vi "terminate.vi"(8 "error in (no error)":errorcluster, 11 "GenericImageProcessor in":refnum<class "GenericImageProcessor.lvclass">) -> (0 "error out":errorcluster, 3 "GenericImageProcessor out":refnum<class "GenericImageProcessor.lvclass">)   [LabVIEW 2010, in "GenericImageProcessor.lvclass"]
uses:
  GenericImageProcessor.lvclass
  GenericImageProcessor.lvclass/GenericImageProcessor.ctl
  common/classes/Image/Image/Image.lvclass
  common/classes/GenericComponent/GenericComponent/GenericComponent.lvclass
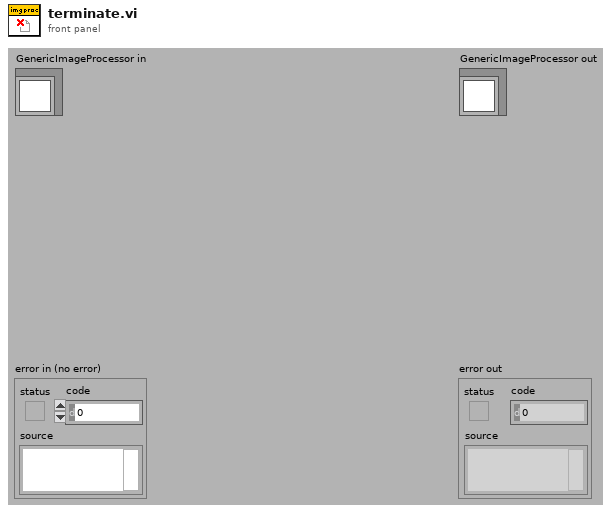
[diagram p1: front panel]
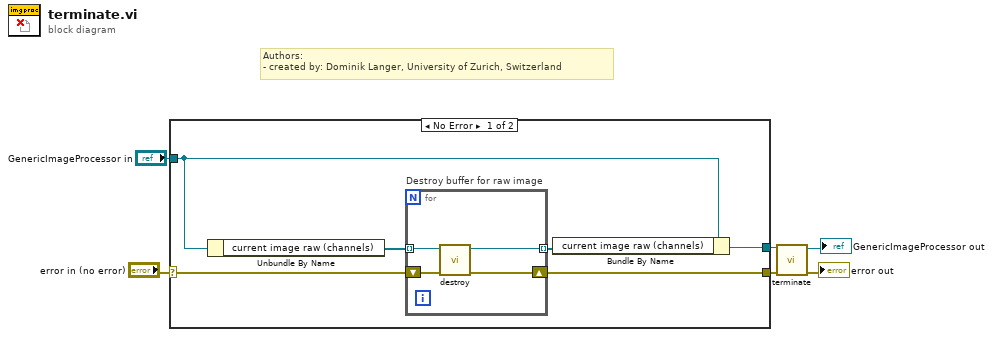
[diagram p0: block diagram]
diagram:
  # "Authors: \n- created by: Dominik Langer, University of Zurich, Switzerland"
  n1 = case shown="No Error" "error in (no error)" {
    selector: "error in (no error)" -> [w12 w18]
    tunnel: [w7 w18] -> w4
    tunnel: [w8 w17] -> w1
    tunnel: "GenericImageProcessor in" -> [w9 w17]
    frame No Error {
      n2 = Unbundle By Name(w9) -> ("current image raw (channels)"=w11:refnum<class "Image.lvclass">[])
      n3 = for "Destroy buffer for raw image" {
        shift-right: [w15] -> w7
        shift-left: w12 -> [w16]
        tunnel: w11 -> [w14] mode=indexing
        tunnel: [w13] -> w10 mode=indexing
        n4 = call-dynamic "destroy.vi"("error in (no error)"=w16, "Image in"=w14) -> ("error out"=w15:errorcluster, "Image out"=w13:refnum<class "Image.lvclass">)  [unwired: 8 out]
      }
      n5 = Bundle By Name(cluster=w9, "current image raw (channels)"=w10) -> (w8:refnum<class "GenericImageProcessor.lvclass">)
    }
    frame Error {
    }
  }
  n6 = call-parent "terminate.vi"("error in (no error)"=w4, "GenericPlugin in"=w1) -> ("error out"=→"error out":errorcluster, "GenericPlugin out"=→"GenericImageProcessor out":refnum<class "GenericImageProcessor.lvclass">)  [unwired: 8 out]
